vi "Set Data.vi"(8 "error in (no error)":errorcluster, 9 "Power":sgl, 10 "T":sgl, 11 "TECData in":refnum<class "TECData.lvclass">) -> (0 "error out":errorcluster, 3 "TECData out":refnum<class "TECData.lvclass">)   [LabVIEW 2018, in "TE Cooler.lvlib" / "TECData.lvclass"]
doc: "Write the data to the instance. Temperature and power are the two variables we will be retrieving and consider the main data."
uses:
  TECData.lvclass
  TECData.lvclass/TECData.ctl
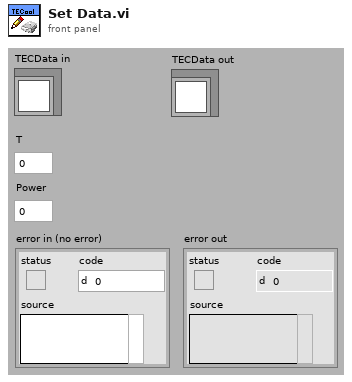
[diagram p1: front panel]
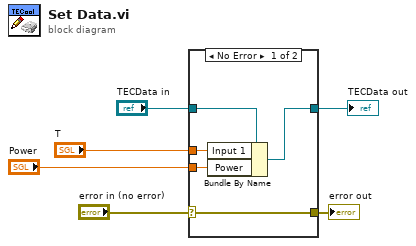
[diagram p0: block diagram]
diagram:
  n1 = case shown="No Error" "error in (no error)" {
    selector: "error in (no error)" -> [w11 w13]
    tunnel: [w11 w13] -> w5
    tunnel: [w9 w12] -> w3
    tunnel: "TECData in" -> [w10 w12]
    tunnel: "T" -> [w8 _]
    tunnel: "Power" -> [w7 _]
    frame No Error {
      n2 = Bundle By Name(cluster=w10, "Input 1"=w8, "Power"=w7) -> (w9:refnum<class "TECData.lvclass">)
    }
    frame Error {
    }
  }
  "error out" <- w5
  "TECData out" <- w3
